vi "Initialize DAQ (Ctr As Clk).vi"(8 "error in (no error)":errorcluster, 10 "DAQ Settings":T2, 11 "DAQmx Resource":tag) -> (0 "error out":errorcluster, 3 "DAQmx Tasks":T1)   [LabVIEW 2025]
uses:
  <vilib>/DAQmx/write.llb/DAQmx Write (Digital Wfm 1Chan NSamp).vi
  <vilib>/DAQmx/create/channels.llb/DAQmx Create Channel (CO-Pulse Generation-Frequency).vi
  <vilib>/DAQmx/configure/timing.llb/DAQmx Timing (Implicit).vi
  <vilib>/Waveform/DWDTOps.llb/DWDT Append Digital Samples.vi
  <vilib>/Waveform/DWDTOps.llb/DWDT Digital Size.vi
  <vilib>/DAQmx/configure/timing.llb/DAQmx Timing (Sample Clock).vi
  <vilib>/Waveform/DWDTOps.llb/DWDT Uncompress Digital.vi
  <vilib>/DAQmx/miscellaneous.llb/DAQmx Fill In Error Info.vi
  <resource>/objmgr/daqmx.rc
panel:
  out "Actual Sample Rate Frequency":dbl
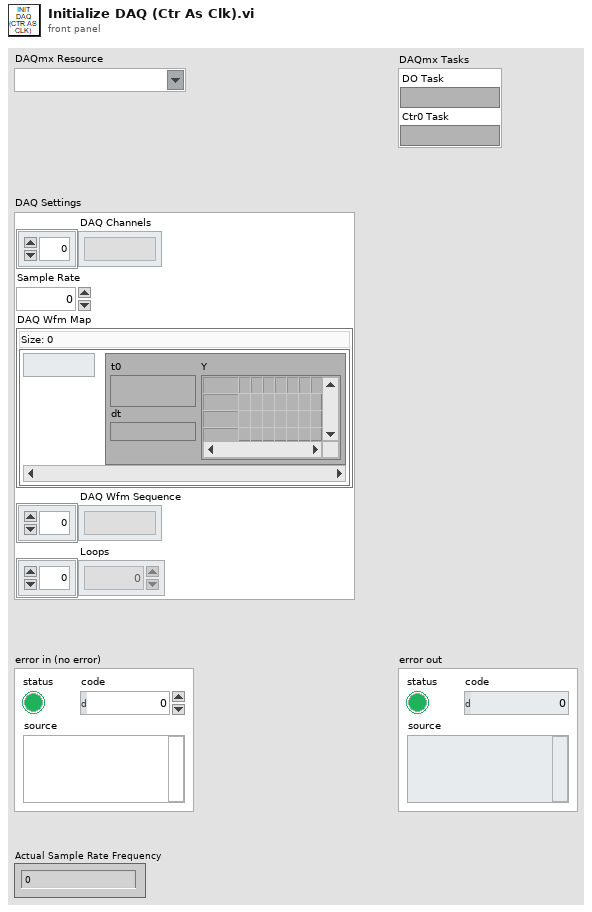
[diagram p1: front panel]
types:
  T1 = cluster{"DO Task":refnum<k21>, "Ctr0 Task":refnum<k21>}
  T2 = cluster{"DAQ Channels":string[], "Sample Rate":dbl, "DAQ Wfm Map":map{string, digitalwaveform}, "DAQ Wfm Sequence":string[], "Loops":i32[]}
  T3 = cluster{"task out":refnum<k21>, "task out":refnum<k21>}
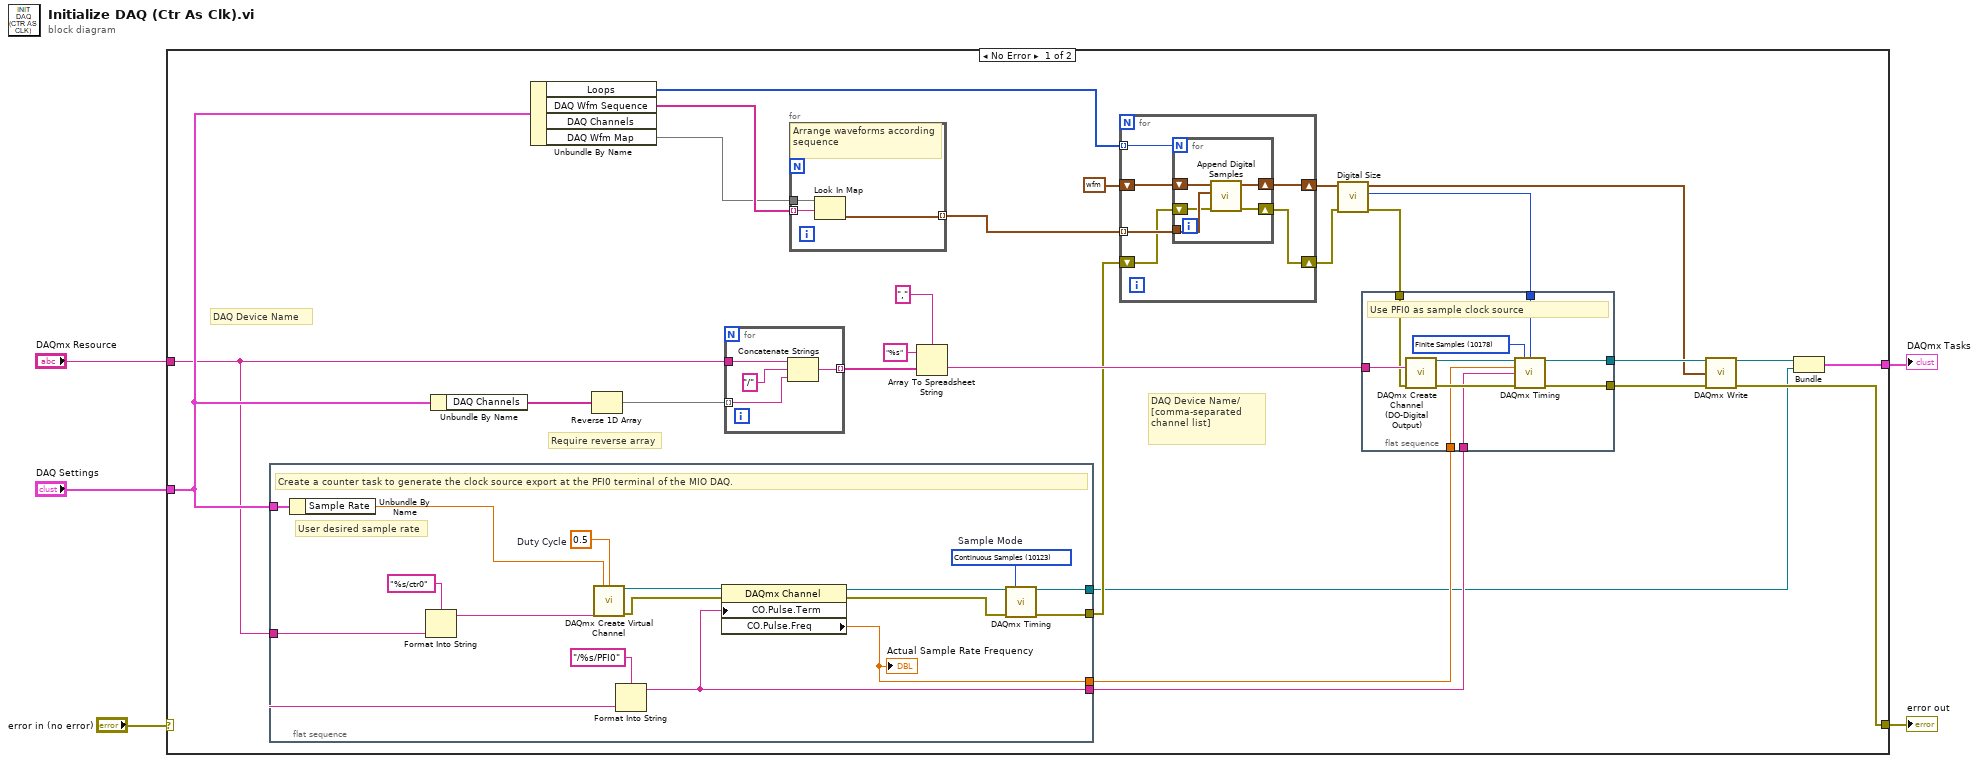
[diagram p0: block diagram]
diagram:
  n1 = case shown="No Error" "error in (no error)" {
    selector: "error in (no error)" -> [_ w77]
    tunnel: [w22 w77] -> w5
    tunnel: "DAQmx Resource" -> [w20 _]
    tunnel: "DAQ Settings" -> [w31 _]
    tunnel: [w11 _] -> w1
    frame No Error {
      # "Require reverse array"
      # "DAQ Device Name/[comma-separated channel list]"
      # "DAQ Device Name"
      n2 = flat-sequence {
        tunnel: w31 -> [w58]
        tunnel: w20 -> [w47]
        tunnel: [w46] -> w19
        tunnel: [w45] -> w14
        tunnel: [w44] -> w18
        tunnel: [w43] -> w10
        frame #0 {
          w52 = 0.5  # Duty Cycle
          w57 = 10123 items=["Finite Samples"=10178, "Continuous Samples"=10123, "Hardware Timed Single Point"=12522]  # Sample Mode
          # "User desired sample rate"
          # "Create a counter task to generate the clock source export at the PFI0 terminal of the MIO DAQ."
          n3 = Unbundle By Name(w58) -> ("Sample Rate"=w51:dbl)
          n4 = Format Into String(format string="%s/ctr0", w47) -> (resulting string=w49:string)  [unwired: 2 in, 1 out]
          n5 = call-poly <vilib>:"DAQmx Create Virtual Channel.vi"("frequency"=w51, "duty cycle"=w52, "counter"=w49) -> ("task out"=w56:refnum<k21>, "error out"=w55:errorcluster)  [unwired: 11 in]
          n6 = Format Into String(format string="/%s/PFI0", w47) -> (resulting string=w44:string)  [unwired: 2 in, 1 out]
          n7 = property class="DAQmx Channel"(reference=w56, error in=w55, "CO.Pulse.Term"=w44) -> (reference out=w53:refnum<k21>, error out=w54:errorcluster, "CO.Pulse.Freq"=w46:dbl)
          "Actual Sample Rate Frequency" <- w46
          n8 = call-poly <vilib>:"DAQmx Timing.vi"("task/channels in"=w53, "sample mode"=w57, "error in"=w54) -> ("task out"=w43:refnum<k21>, "error out"=w45:errorcluster)  [unwired: 11 in]
        }
      }
      n9 = Unbundle By Name(w31) -> ("DAQ Channels"=w30:string[])
      n10 = Unbundle By Name(w31) -> ("Loops"=w9:i32[], "DAQ Wfm Sequence"=w32:string[], "DAQ Wfm Map"=w25:map{string, digitalwaveform})  [unwired: 1 out]
      n11 = Reverse 1D Array(array=w30) -> (reversed array=w6:string[])
      n12 = for {
        tunnel: w20 -> [w76]
        tunnel: w6 -> [w74] mode=indexing
        tunnel: [w73] -> w29 mode=indexing
        n13 = Concatenate Strings(w76, "/", w74) -> (w73:string)
      }
      n14 = for {
        tunnel: w32 -> [w72] mode=indexing
        tunnel: w25 -> [w71]
        tunnel: [w70] -> w24 mode=indexing
        # "Arrange waveforms according sequence"
        n15 = Look In Map(map=w71, key=w72) -> (value=w70:digitalwaveform)  [unwired: 1 in, 1 out]
      }
      n16 = Array To Spreadsheet String(delimiter (Tab)=",", array=w29, 3:"%s" ("format string")) -> (spreadsheet string=w26:string)
      n17 = for {
        shift-right: [w63] -> w17
        shift-left: digitalwaveform {"t0"=timestamp(0 s since 1904-01-01), "dt"=0.0, "Y"={"transitions"=[], "data"=[]}} ("digital waveform out") -> [w64]
        tunnel: w24 -> [w62] mode=indexing
        shift-right: [w60] -> w15
        shift-left: w14 -> [w61]
        tunnel: w9 -> [w59] mode=indexing
        n18 = for {
          N: w59 -> [_]
          tunnel: w62 -> [w67]
          shift-right: [w68] -> w63
          shift-left: w64 -> [w69]
          shift-right: [w65] -> w60
          shift-left: w61 -> [w66]
          n19 = call-poly <vilib>:"Append Digital Samples.vi"("error in (no error)"=w66, "digital waveform B"=w67, "digital waveform A"=w69) -> ("error out"=w65:errorcluster, "digital waveform out"=w68:digitalwaveform)  [unwired: 7 in]
        }
      }
      n20 = call-poly <vilib>:"Digital Size.vi"("error in (no error)"=w15, "digital waveform in"=w17) -> ("error out"=w13:errorcluster, "number of samples"=w16:i32, "digital waveform out"=w7:digitalwaveform)  [unwired: 6 in, 1 out]
      n21 = flat-sequence {
        tunnel: w26 -> [w42]
        tunnel: [w38] -> w21
        tunnel: w19 -> [w37]
        tunnel: w18 -> [w36]
        tunnel: w16 -> [w35]
        tunnel: w13 -> [w34]
        tunnel: [w33] -> w12
        frame #0 {
          w39 = 10178 items=["Finite Samples"=10178, "Continuous Samples"=10123, "Hardware Timed Single Point"=12522] ("sample mode")
          # "Use PFI0 as sample clock source"
          n22 = call <vilib>:"DAQmx Create Channel (DO-Digital Output).vi"("lines"=w42, "error in"=w34) -> ("task out"=w40:refnum<k21>, "error out"=w41:errorcluster)  [unwired: 12 in]
          n23 = call-poly <vilib>:"DAQmx Timing.vi"("task/channels in"=w40, "sample mode"=w39, "samples per channel"=w35, "rate"=w37, "source"=w36, "error in"=w41) -> ("task out"=w38:refnum<k21>, "error out"=w33:errorcluster)  [unwired: 8 in]
        }
      }
      n24 = call-poly <vilib>:"DAQmx Write.vi"("task/channels in"=w21, "data"=w7, "error in"=w12) -> ("task out"=w23:refnum<k21>, "error out"=w22:errorcluster)  [unwired: 10 in, 1 out]
      n25 = Bundle("task out"=w23, "task out"=w10) -> (w11:T3)  [unwired: 1 in]
    }
    frame Error {
    }
  }
  "error out" <- w5
  "DAQmx Tasks" <- w1
